vi "07FootGlobals.vi"() -> ()   [LabVIEW 2020]
panel:
  in  "Data":dbl[](array[numeric])
  in  "DAQState":enum16{"GetData", "StopDAQ", "Quit"}(ring)
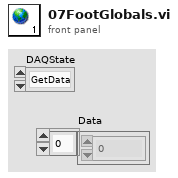
[diagram p1: front panel]
diagram:
